vi "my_solution_plain.vi"() -> ()   [LabVIEW 2013]
doc: "This example performs writes and reads on a serial port, as directed by the user. You can press the Write and Read buttons, and change the Read Count, while the example is running.\n\nThe parameters set for the serial port must match the parameters of the connected instrument or device. In this example, the Read Count parameter specifies the number of bytes that the serial port reads. If there were more bytes at the port than the specified number, those bytes would not be read. If there were less bytes at the port than the specified number, you would receive a timeout error.\n\nThis example expands upon the flow control options for XON and XOFF, allowing the user to choose those control characters. Also, the user can enable or disable a termination character. Some devices require a termination character in order to identify the end of command strings. Some devices send a termination character to signify the end of data to be read. This example shows how you can end the Read operation once a termination character is detected in the buffer and/or append a termination character at the end of the Write data."
uses:
  C:/Program Files (x86)/National Instruments/LabVIEW 2013/examples/Instrument IO/Serial/support/Serial - Settings.ctl
  <vilib>/Instr/_visa.llb/VISA Configure Serial Port (Instr).vi
panel:
  out "Response":string
  out "Waveform Chart 4":T1(graph)
  in  "Stop":bool
  in  "Command":string="*IDN?"
  in  "Read Count":u32=1000
  in  "Write":bool
  in  "Read":bool
  in  "Serial Settings":T2={"baud rate"=115200, "data bits"=8, "parity"=enum."None", "stop bits"=10, "flow control"=0} {"flow control" items=["None"=0, "XON/XOFF"=1, "RTS/CTS"=2, "DTR/DSR"=4]; "stop bits" items=["1.0"=10, "1.5"=15, "2.0"=20]; "data bits" min=5 max=8 step=1; "baud rate" items=["75"=75, "110"=110, "134"=134, "150"=150, "300"=300, "600"=600, "1200"=1200, "1800"=1800, "2400"=2400, "4800"=4800, "7200"=7200, "9600"=9600, "14400"=14400, "19200"=19200, "28800"=28800, "38400"=38400, "56000"=56000, "57600"=57600, "115200"=115200, "128000"=128000, "230400"=230400]}
  in  "VISA resource name":refnum<visa-resource-name>="COM4"
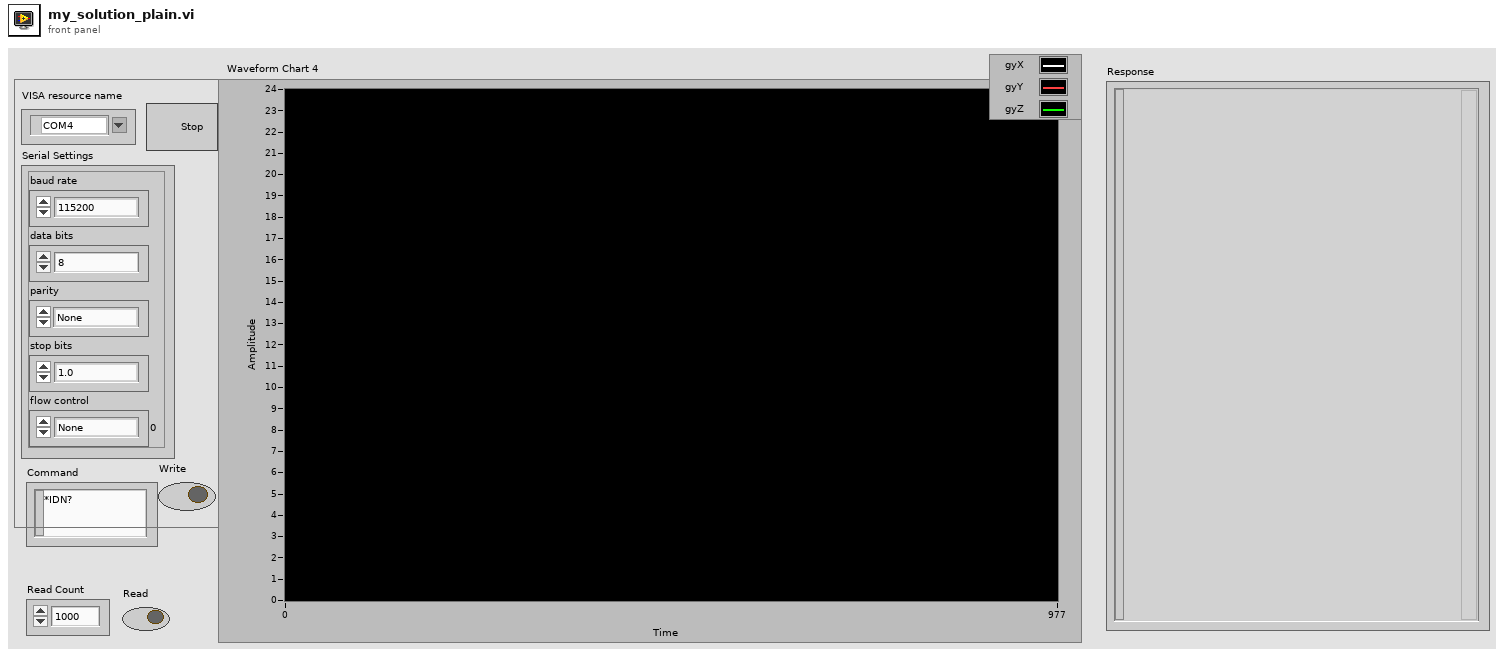
[diagram p1: front panel]
types:
  T1 = cluster{"Numeric Control":dbl, "Numeric Control":dbl, "Numeric Control":dbl}
  T2 = typedef "Serial - Settings.ctl" = cluster{"baud rate":u32, "data bits":u16, "parity":enum16{"None", "Odd", "Even", "Mark", "Space"}, "stop bits":u16, "flow control":u16}
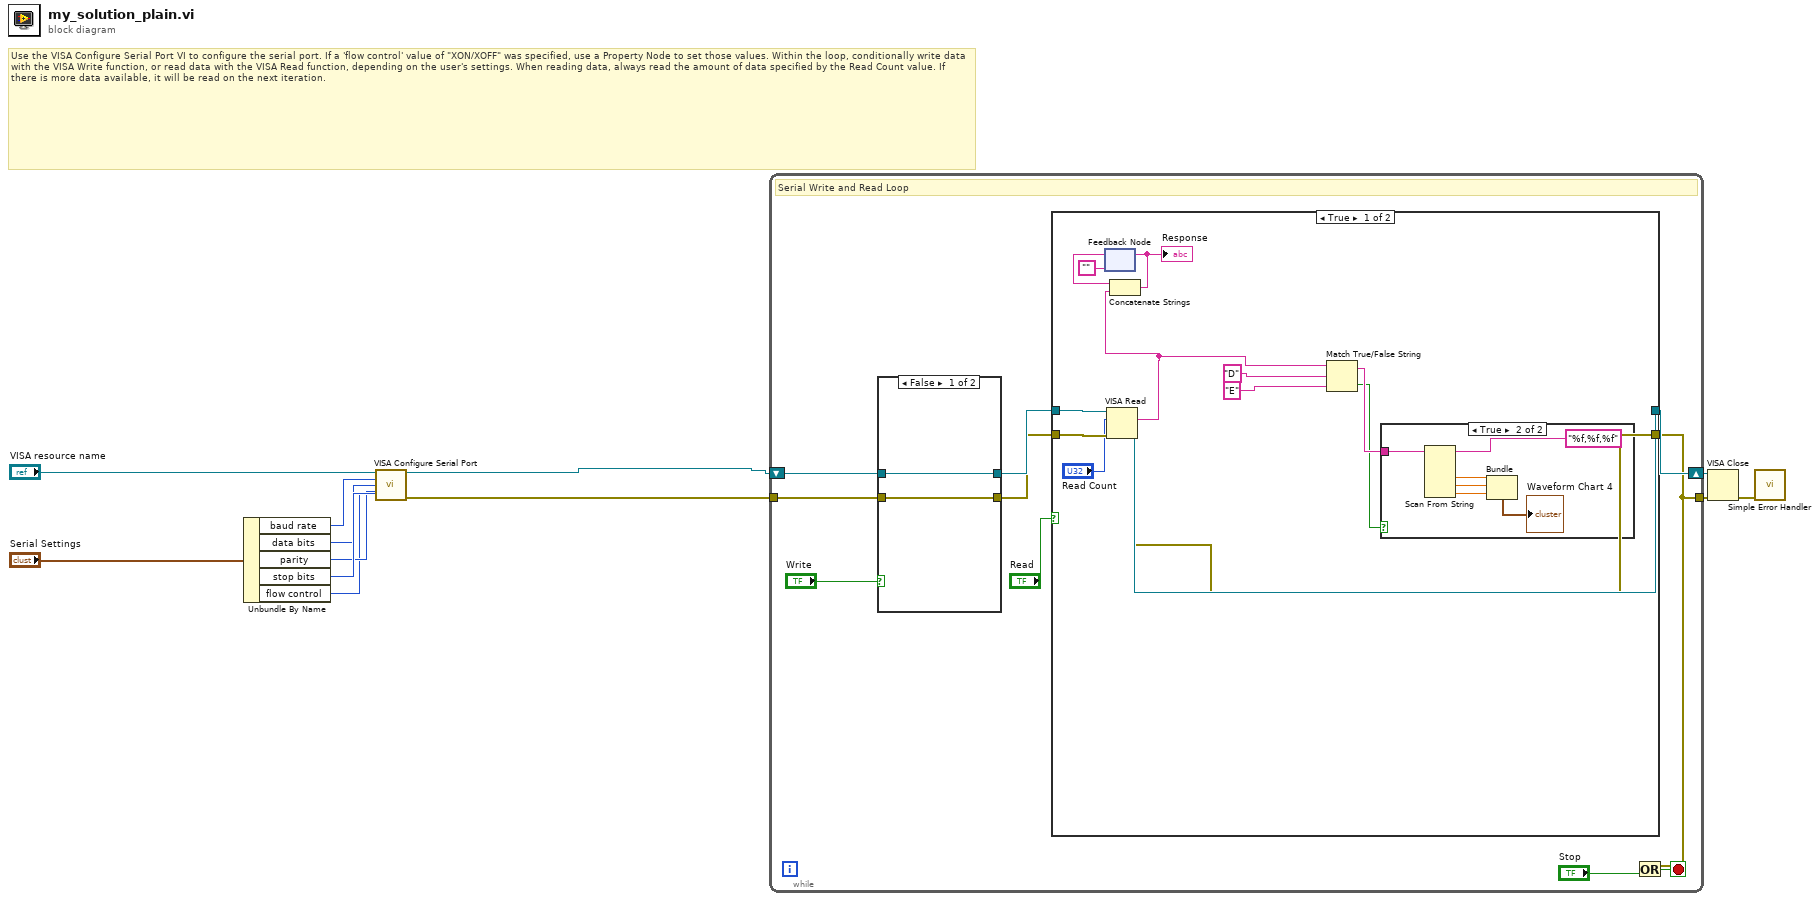
[diagram p0: block diagram]
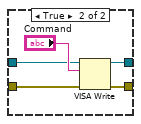
[diagram p2: hidden frame]
diagram:
  # "Use the VISA Configure Serial Port VI to configure the serial port. If a 'flow control' value of \"XON/XOFF\" was specified, use a Property Node to set those values. Within the loop, conditionally write data with the VISA Write function, or read data with the VISA Read function, depending on the user's settings. When reading data, always read the amount of data specified by the Read Count value. If there is more data available, it will be read on the next iteration."
  n1 = Unbundle By Name("Serial Settings") -> ("baud rate"=w8:u32, "data bits"=w9:u16, "parity"=w10:enum16{"None", "Odd", "Even", "Mark", "Space"}, "stop bits"=w11:u16, "flow control"=w3:u16)
  n2 = call-poly "VISA Configure Serial Port"("VISA resource name"="VISA resource name", "baud rate (9600)"=w8, "data bits (8)"=w9, "parity (0:none)"=w10, "stop bits (10: 1 bit)"=w11, "flow control (0:none)"=w3) -> ("VISA resource name out"=w2:refnum<visa-resource-name>, "error out"=w1:errorcluster)  [unwired: 4 in, 4 out]
  n3 = while {
    shift-right: [w22] -> w4
    shift-left: w2 -> [w21]
    tunnel: w1 -> [w20]
    tunnel: [w15] -> w5
    stop <- w16 stop-if-true
    # "Serial Write and Read Loop"
    n4 = case shown="False" "Write" {
      tunnel: w21 -> [w24 w28]
      tunnel: w20 -> [w23 w27]
      tunnel: [w24 w26] -> w19
      tunnel: [w23 w25] -> w18
      frame False {
      }
      frame True {
        n5 = VISA Write(VISA resource name=w28, write buffer="Command", error in (no error)=w27) -> (VISA resource name out=w26:refnum<visa-resource-name>, error out=w25:errorcluster)  [unwired: 1 out]
      }
    }
    n6 = case shown="True" "Read" {
      tunnel: [w40 w50] -> w22
      tunnel: w19 -> [w42 w50]
      tunnel: [w38 w49] -> w15
      tunnel: w18 -> [w41 w49]
      frame True {
        n7 = feedback #1("") -> (w33:string)
        n8 = VISA Read(VISA resource name=w42, byte count="Read Count", error in (no error)=w41) -> (VISA resource name out=w40:refnum<visa-resource-name>, read buffer=w30:string, error out=w38:errorcluster)  [unwired: 1 out]
        n9 = Concatenate Strings(w33, w30) -> (w32:string)
        "Response" <- w32
        n10 = feedback-in #1(w32) -> ()
        n11 = Match True/False String(2:"E" ("false string"), 3:"D" ("true string"), 4:w30) -> (0:w34:bool, 1:w35:string)
        n12 = case shown="True" w34 {
          tunnel: w35 -> [_ w43]
          frame False {
          }
          frame True {
            n13 = Scan From String(format string="%f,%f,%f", input string=w43) -> (output 1=w46:dbl, output 2=w45:dbl, output 3=w44:dbl)  [unwired: 5 in, 3 out]
            n14 = Bundle(w46, w45, w44) -> (→"Waveform Chart 4":cluster{dbl, dbl, dbl})  [unwired: 1 in]
          }
        }
      }
      frame False {
      }
    }
    n15 = Or(x=w15, y="Stop") -> (x .or. y?=w16:bool)
  }
  n16 = VISA Close(VISA resource name=w4, error in (no error)=w5) -> (error out=w6:errorcluster)
  n17 = call <vilib>:"Simple Error Handler.vi"("error in (no error)"=w6) -> ()  [unwired: 1 in, 8 out]
